vi "Obtain Motor Communication Ref.vi"(8 "error in (no error)":errorcluster, 11 "motor name":string) -> (0 "error out":errorcluster, 1 "valid?":bool, 3 "motor communication ref out":refnum<class "NI_Robotics_Motor Communication Ref.lvclass">)   [LabVIEW 2017, in "NI_Robotics_Motor Communication Ref.lvclass"]
doc: "Obtains and existing communication session for a motor."
uses:
  <vilib>/robotics/Actuation/Motor Communication Ref/NI_Robotics_Motor Communication Ref.lvclass
  <vilib>/robotics/Actuation/Motor Communication Ref/FG Motor Comm Ref Sessions Action.ctl
  <vilib>/robotics/Actuation/Motor Communication Ref/NI_Robotics_Motor Communication Ref.lvclass/NI_Robotics_Motor Communication Ref.ctl
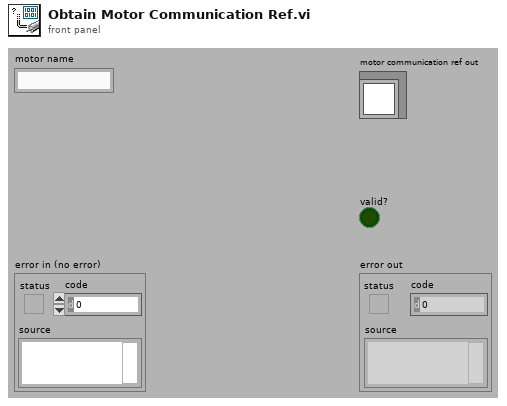
[diagram p1: front panel]
types:
  T1 = typedef "NI_Robotics_Motor Communication Ref.lvclass/FG Motor Comm Ref Sessions Action.ctl" = enum16{"Get", "Add", "Delete"}
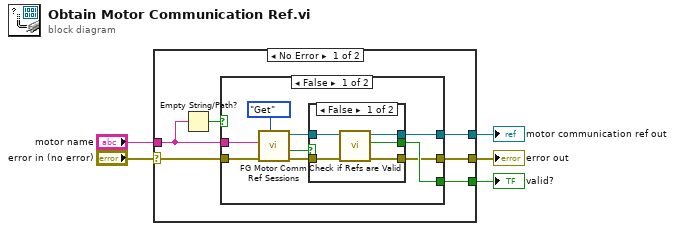
[diagram p0: block diagram]
diagram:
  n1 = case shown="No Error" "error in (no error)" {
    selector: "error in (no error)" -> [w11 w29]
    tunnel: [w9 w29] -> w4
    tunnel: [w8 _] -> w3
    tunnel: "motor name" -> [w7 _]
    tunnel: [w10 _] -> w1
    frame No Error {
      n2 = Empty String/Path?(string/path=w7) -> (empty?=w6:bool)
      n3 = case shown="False" w6 {
        tunnel: w11 -> [w20 w28]
        tunnel: [w16 _] -> w10
        tunnel: [w15 w28] -> w9
        tunnel: [w14 _] -> w8
        tunnel: w7 -> [w13 _]
        frame False {
          n4 = call <vilib>:"FG Motor Comm Ref Sessions.vi"("action"=FG_Motor_Comm_Ref_Sessions_Action."Get", "error in (no error)"=w20, "motor name"=w13) -> ("error out"=w19:errorcluster, "failed?"=w17:bool, "motor communication ref out"=w18:refnum<class "NI_Robotics_Motor Communication Ref.lvclass">)  [unwired: 6 in]
          n5 = case shown="False" w17 {
            tunnel: w18 -> [w25 w26]
            tunnel: [w24 w26] -> w14
            tunnel: w19 -> [w23 w27]
            tunnel: [w21 _] -> w16
            tunnel: [w22 w27] -> w15
            frame False {
              n6 = call <vilib>:"Check if Refs are Valid.vi"("error in (no error)"=w23, "motor communication ref in"=w25) -> ("error out"=w22:errorcluster, "valid?"=w21:bool, "motor communication ref out"=w24:refnum<class "NI_Robotics_Motor Communication Ref.lvclass">)  [unwired: 7 in]
            }
            frame True {
            }
          }
        }
        frame True {
        }
      }
    }
    frame Error {
    }
  }
  "error out" <- w4
  "motor communication ref out" <- w3
  "valid?" <- w1
